vi "Coordinates Next to Each Other (incl diag).vi"(10 "Tail Positions":T1, 11 "Head Position":T1) -> (2 "Neighbouring":bool, 3 "Next to each other":bool)   [LabVIEW 2021]
uses:
  Positions.ctl
panel:
  out "Diagonal":bool
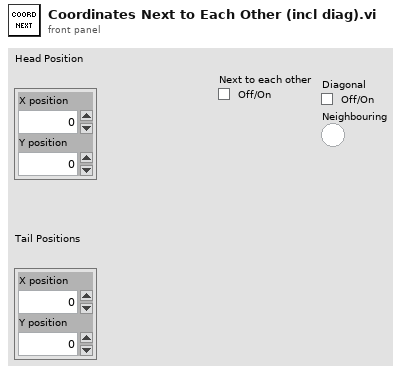
[diagram p1: front panel]
types:
  T1 = typedef "Positions.ctl" = cluster{"X position":i32, "Y position":i32}
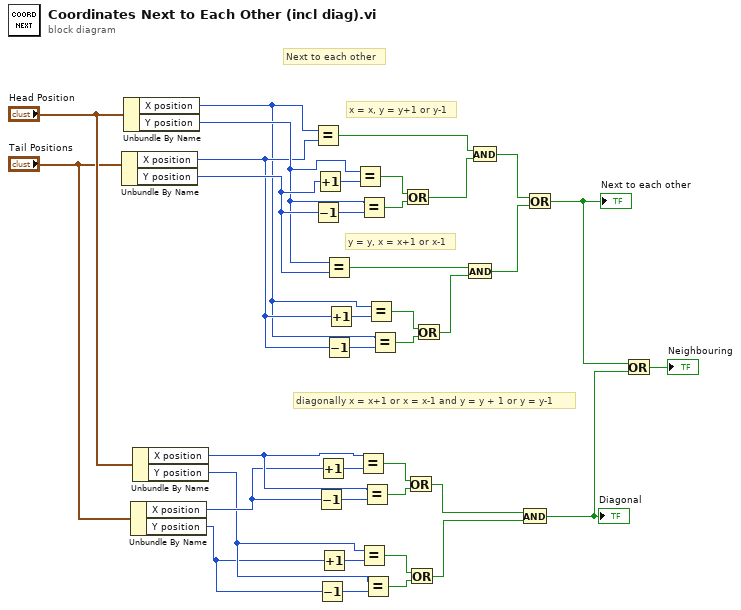
[diagram p0: block diagram]
diagram:
  # "diagonally x = x+1 or x = x-1 and y = y + 1 or y = y-1"
  # "Next to each other"
  # "y = y, x = x+1 or x-1"
  # "x = x, y = y+1 or y-1"
  n1 = Unbundle By Name("Tail Positions") -> ("X position"=w24:i32, "Y position"=w33:i32)
  n2 = Unbundle By Name("Head Position") -> ("X position"=w23:i32, "Y position"=w32:i32)
  n3 = Unbundle By Name("Tail Positions") -> ("X position"=w8:i32, "Y position"=w6:i32)
  n4 = Unbundle By Name("Head Position") -> ("X position"=w9:i32, "Y position"=w7:i32)
  n5 = Equal?(x=w23, y=w24) -> (x = y?=w37:bool)
  n6 = Decrement(x=w33) -> (x-1=w34:i32)
  n7 = Increment(x=w33) -> (x+1=w35:i32)
  n8 = Decrement(x=w8) -> (x-1=w15:i32)
  n9 = Decrement(x=w6) -> (x-1=w11:i32)
  n10 = Increment(x=w8) -> (x+1=w16:i32)
  n11 = Increment(x=w6) -> (x+1=w12:i32)
  n12 = Equal?(x=w32, y=w33) -> (x = y?=w29:bool)
  n13 = Decrement(x=w24) -> (x-1=w26:i32)
  n14 = Increment(x=w24) -> (x+1=w27:i32)
  n15 = Equal?(x=w32, y=w35) -> (x = y?=w31:bool)
  n16 = Equal?(x=w9, y=w16) -> (x = y?=w14:bool)
  n17 = Equal?(x=w32, y=w34) -> (x = y?=w36:bool)
  n18 = Equal?(x=w7, y=w12) -> (x = y?=w10:bool)
  n19 = Equal?(x=w9, y=w15) -> (x = y?=w17:bool)
  n20 = Equal?(x=w7, y=w11) -> (x = y?=w13:bool)
  n21 = Equal?(x=w23, y=w27) -> (x = y?=w25:bool)
  n22 = Equal?(x=w23, y=w26) -> (x = y?=w28:bool)
  n23 = Or(x=w31, y=w36) -> (x .or. y?=w30:bool)
  n24 = Or(x=w14, y=w17) -> (x .or. y?=w5:bool)
  n25 = Or(x=w10, y=w13) -> (x .or. y?=w4:bool)
  n26 = Or(x=w25, y=w28) -> (x .or. y?=w22:bool)
  n27 = And(x=w29, y=w22) -> (x .and. y?=w20:bool)
  n28 = And(x=w37, y=w30) -> (x .and. y?=w21:bool)
  n29 = And(x=w5, y=w4) -> (x .and. y?=w3:bool)
  "Diagonal" <- w3
  n30 = Or(x=w21, y=w20) -> (x .or. y?=w2:bool)
  "Next to each other" <- w2
  n31 = Or(x=w2, y=w3) -> (x .or. y?=→"Neighbouring":bool)
